vi "Handle setAllData.vi"(8 "error in (no error)":errorcluster, 10 "AllData":variant, 11 "Inst.Krohn-Hite-7008 in":refnum<class "Inst.Krohn-Hite-7008.lvclass">) -> (0 "error out":errorcluster, 3 "Inst.Krohn-Hite-7008 out":refnum<class "Inst.Krohn-Hite-7008.lvclass">)   [LabVIEW 2019, in "Inst.KH7008.lvlib" / "Inst.Krohn-Hite-7008.lvclass"]
doc: "Override to handle \"getAll\" or \"getAllData\" commands for <b>your</b> Instrument"
uses:
  Inst.Krohn-Hite-7008.lvclass
  Inst.Krohn-Hite-7008.lvclass/Inst.Krohn-Hite-7008.ctl
  9f66dee2-c4c4-4da2-ba7b-74040d5a5229.vi
  9f66dee2-c4c4-4da2-ba7b-74040d5a5229.vi/2f7fb02a-5b50-4ae6-8eea-3da043fd12e7.vi
  9f66dee2-c4c4-4da2-ba7b-74040d5a5229.vi/d713c008-804f-468a-bf7d-146784756928.vi
  <vilib>/Utility/Data Type/Get Type Information.vi
  <vilib>/JDP Science/JSONtext/JSON text to Variant.vi
  <vilib>/JDP Science/JSONtext/LVClass Serializer/JSONtext LVClass Serializer.lvclass
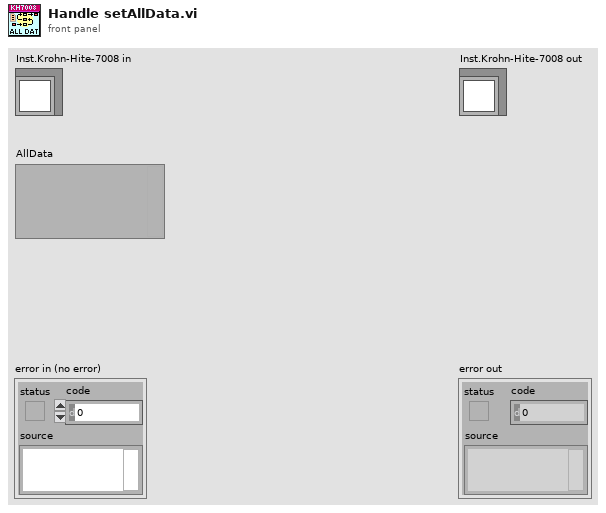
[diagram p1: front panel]
types:
  T1 = typedef "Inst.KH7008.lvlib/Inst.Krohn-Hite-7008.lvclass/Inst.KH7008.getAll--Cluster.ctl" = cluster{"allChannelProperties":T2}
  T2 = typedef "KH7008.lvlib/allChannelProperties--Array.ctl" = T3[]
  T3 = typedef "KH7008.lvlib/channelProperties--Cluster.ctl" = cluster{"channel":T4, "gain":T5, "input":T6, "shunt":T7, "couple":T8, "filter":T9}
  T4 = typedef "KH7008.lvlib/channel--numeric.ctl" = u16
  T5 = typedef "KH7008.lvlib/gain--enum.ctl" = enum16{"1", "10", "100", "1000"}
  T6 = typedef "KH7008.lvlib/input--enum.ctl" = enum16{"OFF", "SE+", "SE-", "DIFF"}
  T7 = typedef "KH7008.lvlib/shunt--enum.ctl" = enum16{"Open", "50", "500", "5k", "50k", "10M"}
  T8 = typedef "KH7008.lvlib/couple--enum.ctl" = enum16{"AC", "DC"}
  T9 = typedef "KH7008.lvlib/filter--enum.ctl" = enum16{"OFF", "ON"}
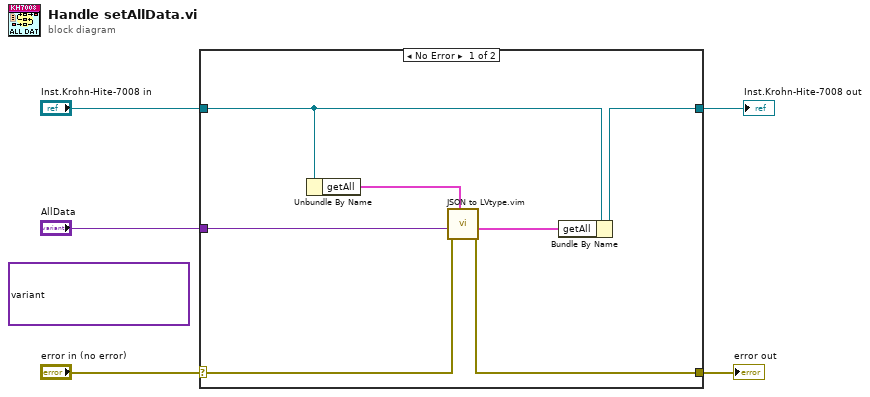
[diagram p0: block diagram]
diagram:
  (unwired) variant(cluster{"channel":u16, "gain":enum16{"1", "10", "100", "1000"}, "input":enum16{"OFF", "SE+", "SE-", "DIFF"}, "shunt":enum16{"Open", "50", "500", "5k", "50k", "10M"}, "couple":enum16{"AC", "DC"}, "filter":enum16{"OFF", "ON"}}[] [{"channel"=1, "gain"=enum."10", "input"=enum."DIFF", "shunt"=enum."50k", "couple"=enum."DC", "filter"=enum."OFF"}, {"channel"=2, "gain"=enum."100", "input"=enum."DIFF", "shunt"=enum."500", "couple"=enum."AC", "filter"=enum."ON"}]) ("AllData")
  n1 = case shown="No Error" "error in (no error)" {
    selector: "error in (no error)" -> [w9 w14]
    tunnel: [w8 w14] -> w3
    tunnel: [w12 w13] -> w4
    tunnel: "Inst.Krohn-Hite-7008 in" -> [w11 w13]
    tunnel: "AllData" -> [w6 _]
    frame No Error {
      n2 = Unbundle By Name(w11) -> ("getAll"=w7:T1)
      n3 = call "JSON to LVtype.vim"("type"=w7, "error in (no error)"=w9, "JSON Data in"=w6) -> ("error out"=w8:errorcluster, "Data out"=w10:T1)  [unwired: 7 in]
      n4 = Bundle By Name(cluster=w11, "getAll"=w10) -> (w12:refnum<class "Inst.Krohn-Hite-7008.lvclass">)
    }
    frame Error {
    }
  }
  "error out" <- w3
  "Inst.Krohn-Hite-7008 out" <- w4
